vi "ANC300_Stop.vi"(0 "ANC300 Communication Port In":refnum<visa-resource-name>, 1 "connection ID in":refnum<k5>, 2 "Axis":u8=1 min=1 max=7, 5 "error in":T1) -> (12 "command string":string, 13 "data out":string, 14 "ANC300 Communication Port Out":refnum<visa-resource-name>, 15 "connection ID out":refnum<k5>, 16 "Axis out":u8=1 min=1 max=7, 18 "transfer ok":bool, 19 "error out":T1)   [LabVIEW 2022 SP3]
panel:
  in  "Time to wait [ms]":u32=200
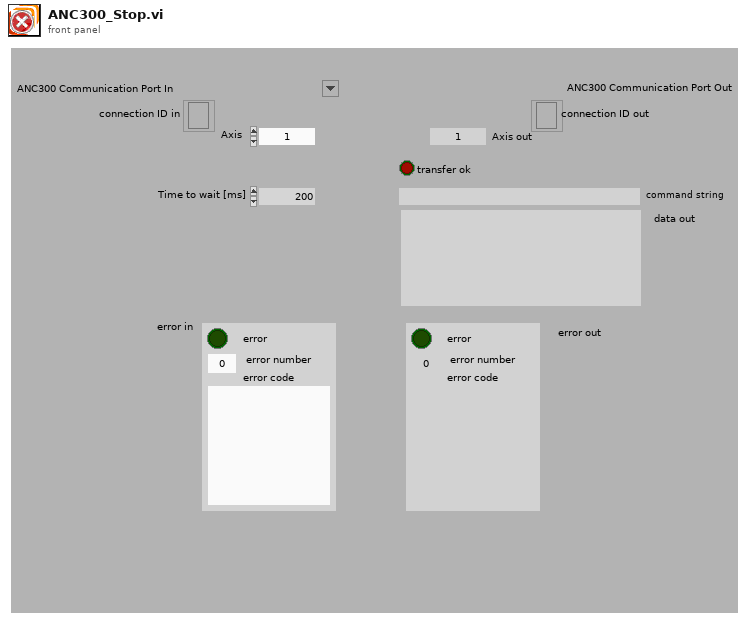
[diagram p1: front panel]
types:
  T1 = cluster{"error ":bool, "error number":i32, "error code":string}
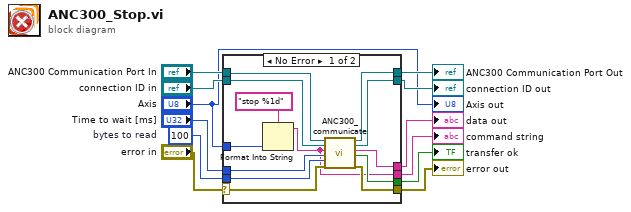
[diagram p0: block diagram]
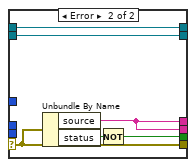
[diagram p2: hidden frame]
diagram:
  w9 = 100  # bytes to read
  n1 = case shown="No Error" "error in" {
    selector: "error in" -> [w18 w29]
    tunnel: "Axis" -> [w13 _]
    tunnel: "ANC300 Communication Port In" -> [w25 w31]
    tunnel: "connection ID in" -> [w24 w30]
    tunnel: "Time to wait [ms]" -> [w23 _]
    tunnel: w9 -> [w22 _]
    tunnel: [w21 w29] -> w3
    tunnel: [w20 w31] -> w7
    tunnel: [w19 w30] -> w6
    tunnel: [w17 w27] -> w2
    tunnel: [w14 w26] -> w5
    tunnel: [w16 w26] -> w4
    frame No Error {
      n2 = Format Into String(format string="stop %1d", w13) -> (resulting string=w14:string)  [unwired: 2 in, 1 out]
      n3 = call "ANC300_communicate.vi"("ANC300 Communication Port In"=w25, "connection ID in"=w24, "commando string"=w14, "Time to wait [ms]"=w23, "bytes to read"=w22, "error in"=w18) -> ("ANC300 Communication Port Out"=w20:refnum<visa-resource-name>, "connection ID out"=w19:refnum<k5>, "read data"=w16:string, "transfer ok"=w17:bool, "error out"=w21:T1)  [unwired: 9 in]
    }
    frame Error {
      n4 = Unbundle By Name(w29) -> ("source"=w26:string, "status"=w28:bool)
      n5 = Not(x=w28) -> (.not. x?=w27:bool)
    }
  }
  "data out" <- w4
  "connection ID out" <- w6
  "error out" <- w3
  "command string" <- w5
  "transfer ok" <- w2
  "ANC300 Communication Port Out" <- w7
  "Axis out" <- "Axis"
